vi "Read Autonomous Moves.vi"() -> ()   [LabVIEW 2012]
doc: "<B>Read Autonomous Moves</B> reads in a text file with a set of moves for the robot and executes those moves. \n\nThe text file must be in the following format:\nLine 1- X Joystick Value (double)\nLine 2- Y Joystick Value (double)\nLine 3- Movement Name (string of either \"right\", \"left\", \"forward\", \"reverse\", or \"stop\")\nLine 4- Encoder Ticks (double)\nLine 5- Empty\nRepeat"
uses:
  <vilib>/Rock Robotics/SystemInterfaces/DIO/FPGA_DIOChannel.ctl
  <vilib>/Rock Robotics/SystemInterfaces/DIO/FPGA_DIOPWMChannel.ctl
  <vilib>/Rock Robotics/SystemInterfaces/Typedef/FPGA_TypedefDigitalModule.ctl
  <vilib>/Rock Robotics/WPI/Counter/WPI_CounterDigitalInputToDigitalSource.vi
  <vilib>/Rock Robotics/WPI/RobotDrive/WPI_RobotDriveOpen2MotorWithJaguar.vi
  <vilib>/Rock Robotics/WPI/RobotDrive/WPI_RobotDriveArcadeDrive_Standard(NoSaturation).vi
  <vilib>/Rock Robotics/WPI/RobotDrive/WPI_RobotDriveArcadeDrive_RatioCurve.vi
panel:
  in  "Movement File Path":path=path "C:/RobotMoves.txt"
  in  "Right Motor (PWM Channel)":T1=enum."PWM 2"
  in  "Left Motor (PWM Channel)":T1
  in  "Encoder Channel 2":T2=enum."DIO 4"
  in  "Encoder Channel 1":T2=enum."DIO 3"
  # "Set these inputs before running."
  # "Wiring Diagram for Digital Sidecar connected to an NI 9403 in slot 4"
  # "Digital Sidecar"
  # "Power\nTerminals"
  # "Motor\nTerminals"
  # "PWM cable"
  # "This shows wiring for a Luminary Micro Jaguar speed controller.  The wiring is similar for a Victor speed controller.  For a Victor, you must also select the appropriate instance of the Motor Open VI on the diagram.  This is only the wiring for the Left Motor.  The Right Motor would be similarly wired to PWM Channel 2."
  # "Wiring Diagram for Digital Sidecar connected to an NI 9403"
  # "This shows wiring for a generic quadrature encoder.  Some encoders may have Gnd labeled as Com.  Some may have +5V labeled as +VDC."
  # "PWR"
  # "SIG"
  # "(-)"
  # "14\n13\n12\n11\n10\n9\n8\n7\n6\n5\n4\n3\n2\n1"
  # "Encoder"
  # "DIGITAL I/O"
  # "Index"
  # "Gnd"
  # "+5V"
  # "B"
  # "A"
  # "Digital Sidecar"
  # "PWR"
  # "SIG"
  # "(-)"
  # "+V"
  # "10"
  # "9"
  # "8"
  # "7"
  # "6"
  # "5"
  # "4"
  # "3"
  # "2"
  # "1"
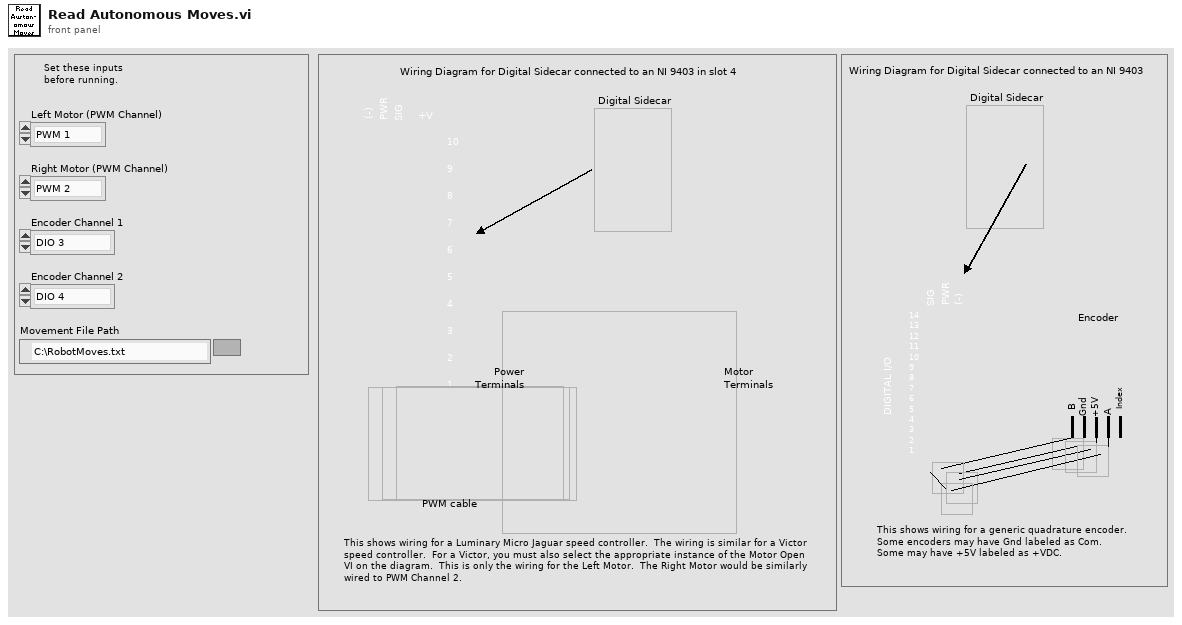
[diagram p1: front panel]
types:
  T1 = typedef "FPGA_DIOPWMChannel.ctl" = enum8{"PWM 1", "PWM 2", "PWM 3", "PWM 4", "PWM 5", "PWM 6", "PWM 7", "PWM 8", "PWM 9", "PWM 10", "Invalid"}
  T2 = typedef "FPGA_DIOChannel.ctl" = enum8{"DIO 1", "DIO 2", "DIO 3", "DIO 4", "DIO 5", "DIO 6", "DIO 7", "DIO 8", "DIO 9", "DIO 10", "DIO 11", "DIO 12", "DIO 13", "DIO 14", "Invalid"}
  T3 = typedef "FPGA_TypedefDigitalModule.ctl" = enum16{"Digital Module 1", "Digital Module 2"}
  T4 = typedef "WPI_DigitalInputDevRef.ctl" = cluster{"DevStatus":errorcluster, "DIO Channel":T2, "Digital Module":T3}
  T5 = typedef "FPGA_CounterEncoderSourceConvertionLVSourceType.ctl" = cluster{"DevStatus":errorcluster, "AnalogTriggerMode?":bool, "DigitalMode":cluster{"Digital Module":T3, "DIO Channel":T6}, "AnalogTriggerMode":cluster{"AnalogTriggerIndex":T7, "OutputType":T8}}
  T6 = typedef "FPGA_DIODigitalSourceChannel.ctl" = enum8{"DIO 1", "DIO 2", "DIO 3", "DIO 4", "DIO 5", "DIO 6", "DIO 7", "DIO 8", "DIO 9", "DIO 10", "DIO 11", "DIO 12", "DIO 13", "DIO 14", "Disabled"}
  T7 = typedef "FPGA_AnalogTriggerIndex.ctl" = enum8{"Trig 0", "Trig 1", "Trig 2", "Trig 3", "Trig 4", "Trig 5", "Trig 6", "Trig 7", "Invalid"}
  T8 = typedef "FPGA_AnalogTriggerOutType.ctl" = enum16{"InWindow", "TriggerState", "Rising", "Falling"}
  T9 = typedef "WPI_RobotDriveDevRef.ctl" = cluster{"DevStatus":errorcluster, "Motors[]":T10[], "Square Inputs":bool, "Max Output":dbl, "Isochronous":bool}
  T10 = typedef "WPI_MotorControlDeviceRef.ctl" = cluster{"DeviceStatus":errorcluster, "Type":enum16{"PWM", "CAN"}, "PWM":cluster{"Digital Module":T3, "PWM Channel":T1, "DeadBand":T11}, "CAN":cluster{"Device Number":u8, "Control Mode":T12, "Semaphore":T13, "Max Vout":dbl}, "Invert":bool, "TransformRef":T14, "InvTransformRef":T14}
  T11 = typedef "WPI_PWMDeadband.ctl" = cluster{"Name":string, "maxPositivePwm":i32, "minPositivePwm":i32, "centerPwm":i32, "maxNegativePwm":i32, "minNegativePwm":i32, "angularRange":u16}
  T12 = typedef "WPI_CANJaguar_ControlMode.ctl" = enum8{"Percent VBus", "Current", "Speed", "Position", "Voltage"}
  T13 = typedef "Semaphore RefNum" = refnum<k1>
  T14 = typedef "WPI_PWMTransform_ConPane.ctl" = refnum<vi>
  T15 = typedef "WPI_EncoderDevRef.ctl" = cluster{"DevStatus":errorcluster, "EncoderIndex":T16, "CounterIndex":T17, "DistancePerCount":dbl, "Decoding Type":T18}
  T16 = typedef "FPGA_EncoderIdx.ctl" = enum8{"Enc 0", "Enc 1", "Enc 2", "Enc 3", "Invalid"}
  T17 = typedef "FPGA_CounterCtrSystemIndex.ctl" = enum8{"Ctr 0", "Ctr 1", "Ctr 2", "Ctr 3", "Ctr 4", "Ctr 5", "Ctr 6", "Ctr 7", "Invalid"}
  T18 = typedef "WPI_EncoderType.ctl" = enum16{"1x", "2x", "4x"}
  T19 = cluster{"X Joystick Value":dbl, "Y Joystick Value":dbl, "Movement Name":string, "Ticks":dbl}[]
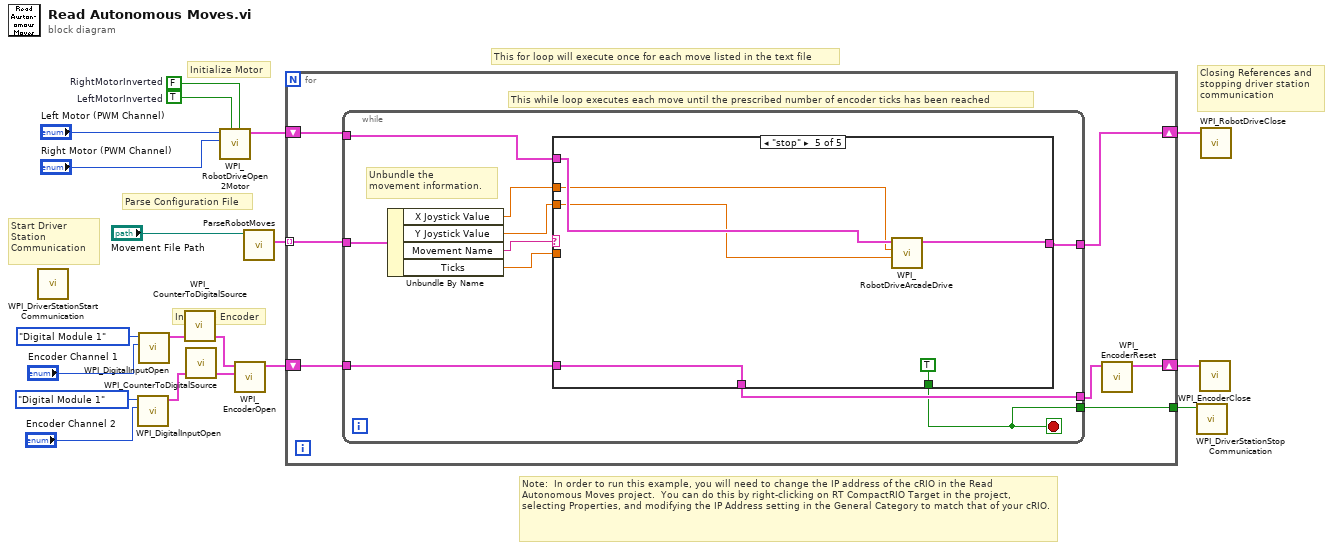
[diagram p0: block diagram]
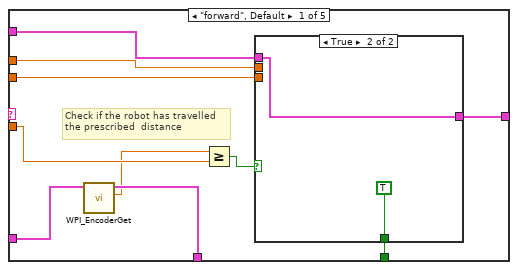
[diagram p2: hidden frame]
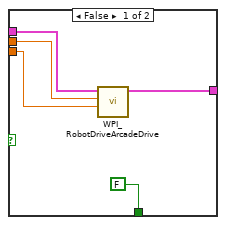
[diagram p3: hidden frame]
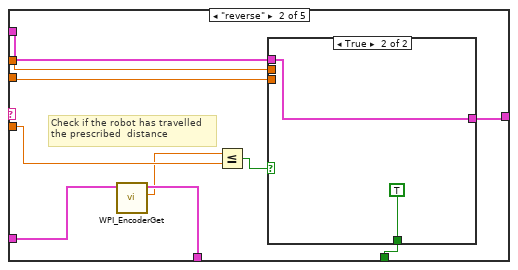
[diagram p4: hidden frame]
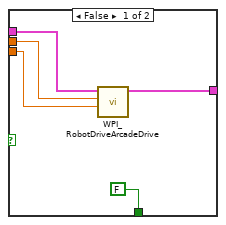
[diagram p5: hidden frame]
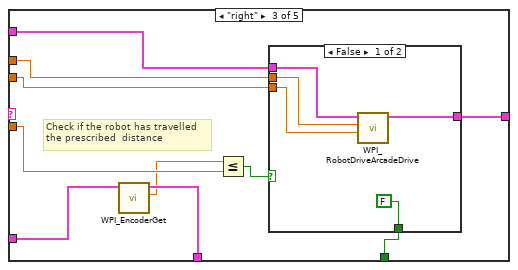
[diagram p6: hidden frame]
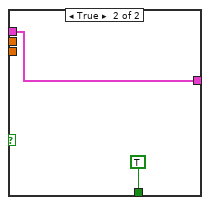
[diagram p7: hidden frame]
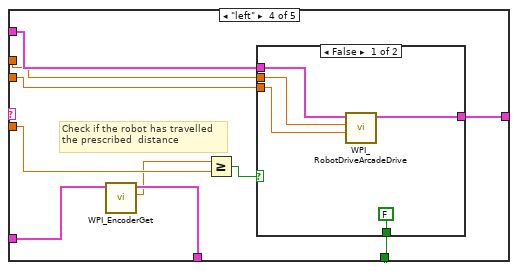
[diagram p8: hidden frame]
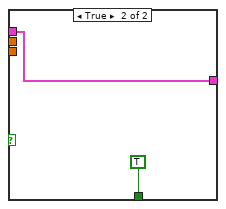
[diagram p9: hidden frame]
diagram:
  w7 = TRUE  # LeftMotorInverted
  w8 = FALSE  # RightMotorInverted
  # "Note:  In order to run this example, you will need to change the IP address of the cRIO in the Read Autonomous Moves project.  You can do this by right-clicking on RT CompactRIO Target in the project, selecting Properties, and modifying the IP Address setting in the General Category to match that of your cRIO."
  # "This for loop will execute once for each move listed in the text file"
  # "Start Driver\nStation \nCommunication"
  # "Closing References and\nstopping driver station\ncommunication"
  # "Parse Configuration File"
  # "Initialize Encoder"
  # "Initialize Motor"
  n1 = call <vilib>:"WPI_DriverStationStart Communication.vi"() -> ()  [unwired: 12 in]
  n2 = call <vilib>:"WPI_DigitalInputOpen.vi"("DIO Channel"="Encoder Channel 2", "Digital Module (Module 1)"=FPGA_TypedefDigitalModule."Digital Module 1") -> ("DigitalInputDevRef"=w16:T4)  [unwired: 8 in, 1 out]
  n3 = call <vilib>:"WPI_DigitalInputOpen.vi"("DIO Channel"="Encoder Channel 1", "Digital Module (Module 1)"=FPGA_TypedefDigitalModule."Digital Module 1") -> ("DigitalInputDevRef"=w17:T4)  [unwired: 8 in, 1 out]
  n4 = call-poly <vilib>:"WPI_CounterToDigitalSource.vi"("DigitalInputDevRef"=w17) -> ("Digital Source"=w14:T5)  [unwired: 6 in]
  n5 = call-poly <vilib>:"WPI_CounterToDigitalSource.vi"("DigitalInputDevRef"=w16) -> ("Digital Source"=w15:T5)  [unwired: 6 in]
  n6 = call-poly <vilib>:"WPI_RobotDriveOpen2Motor.vi"("Right Motor Inverted"=w8, "Left Motor Inverted"=w7, "Right Motor"="Right Motor (PWM Channel)", "Left Motor"="Left Motor (PWM Channel)") -> ("RobotDriveDevRef"=w4:T9)  [unwired: 1 in, 6 out]
  n7 = call <vilib>:"WPI_EncoderOpen.vi"("BSource"=w15, "ASource"=w14) -> ("EncoderDevRef"=w9:T15)  [unwired: 8 in, 1 out]
  n8 = call "ParseRobotMoves.vi"("file path (dialog if empty)"="Movement File Path") -> ("Array"=w18:T19)  [unwired: 10 in]
  n9 = for {
    tunnel: w18 -> [w23] mode=indexing
    shift-right: [w22] -> w2
    shift-left: w4 -> [w21]
    shift-right: [w24] -> w3
    shift-left: w9 -> [w26]
    tunnel: [w20] -> w1
    # "This while loop executes each move until the prescribed number of encoder ticks has been reached"
    n10 = while {
      tunnel: w21 -> [w36]
      tunnel: [w35] -> w22
      tunnel: w26 -> [w29]
      tunnel: [w28] -> w25
      tunnel: w23 -> [w34]
      tunnel: [w27] -> w20
      stop <- w27 stop-if-true
      # "Unbundle the \nmovement information."
      n11 = Unbundle By Name(w34) -> ("X Joystick Value"=w30:dbl, "Y Joystick Value"=w32:dbl, "Movement Name"=w33:string, "Ticks"=w31:dbl)
      n12 = case shown="\"stop\"" w33 {
        tunnel: w36 -> [w44 w62 w79 w95 w110]
        tunnel: w30 -> [w40 w61 w78 w91 w109]
        tunnel: w32 -> [w43 w60 w77 w94 w108]
        tunnel: w31 -> [w46 w59 w76 w93 _]
        tunnel: [w42 w57 w74 w96 w107] -> w35
        tunnel: [w41 w58 w75 w92 TRUE] -> w27
        tunnel: w29 -> [w39 w56 w73 w90 w105]
        tunnel: [w38 w55 w72 w89 w105] -> w28
        frame "forward", Default {
          # "Check if the robot has travelled\nthe prescribed  distance"
          n13 = call <vilib>:"WPI_EncoderGet.vi"("EncoderDevRef"=w39) -> ("Distance"=w37:dbl, "EncoderDevRef"=w38:T15)  [unwired: 5 in, 4 out]
          n14 = Greater Or Equal?(x=w37, y=w46) -> (x >= y?=w45:bool)
          n15 = case shown="True" w45 {
            tunnel: w44 -> [w51 w53]
            tunnel: w43 -> [w50 _]
            tunnel: [w49 w53] -> w42
            tunnel: [FALSE TRUE] -> w41
            tunnel: w40 -> [w47 _]
            frame False {
              n16 = call-poly <vilib>:"WPI_RobotDriveArcadeDrive.vi"("Y axis value"=w50, "X axis value"=w47, "RobotDriveDevRef"=w51) -> ("RobotDriveDevRef"=w49:T9)  [unwired: 1 in, 7 out]
            }
            frame True {
            }
          }
        }
        frame "reverse" {
          # "Check if the robot has travelled\nthe prescribed  distance"
          n17 = call <vilib>:"WPI_EncoderGet.vi"("EncoderDevRef"=w56) -> ("Distance"=w54:dbl, "EncoderDevRef"=w55:T15)  [unwired: 5 in, 4 out]
          n18 = Less Or Equal?(x=w54, y=w59) -> (x <= y?=w63:bool)
          n19 = case shown="True" w63 {
            tunnel: w62 -> [w68 w70]
            tunnel: w61 -> [w67 _]
            tunnel: w60 -> [w66 _]
            tunnel: [w65 w70] -> w57
            tunnel: [FALSE TRUE] -> w58
            frame False {
              n20 = call-poly <vilib>:"WPI_RobotDriveArcadeDrive.vi"("Y axis value"=w66, "X axis value"=w67, "RobotDriveDevRef"=w68) -> ("RobotDriveDevRef"=w65:T9)  [unwired: 1 in, 7 out]
            }
            frame True {
            }
          }
        }
        frame "right" {
          # "Check if the robot has travelled\nthe prescribed  distance"
          n21 = call <vilib>:"WPI_EncoderGet.vi"("EncoderDevRef"=w73) -> ("Distance"=w71:dbl, "EncoderDevRef"=w72:T15)  [unwired: 5 in, 4 out]
          n22 = Less Or Equal?(x=w71, y=w76) -> (x <= y?=w80:bool)
          n23 = case shown="False" w80 {
            tunnel: w79 -> [w85 w87]
            tunnel: w78 -> [w84 _]
            tunnel: w77 -> [w83 _]
            tunnel: [w82 w87] -> w74
            tunnel: [FALSE TRUE] -> w75
            frame False {
              n24 = call-poly <vilib>:"WPI_RobotDriveArcadeDrive.vi"("Y axis value (Speed)"=w83, "X axis value (Curve)"=w84, "RobotDriveDevRef"=w85) -> ("RobotDriveDevRef"=w82:T9)  [unwired: 2 in, 6 out]
            }
            frame True {
            }
          }
        }
        frame "left" {
          # "Check if the robot has travelled\nthe prescribed  distance"
          n25 = call <vilib>:"WPI_EncoderGet.vi"("EncoderDevRef"=w90) -> ("Distance"=w88:dbl, "EncoderDevRef"=w89:T15)  [unwired: 5 in, 4 out]
          n26 = Greater Or Equal?(x=w88, y=w93) -> (x >= y?=w97:bool)
          n27 = case shown="False" w97 {
            tunnel: w95 -> [w102 w104]
            tunnel: w91 -> [w101 _]
            tunnel: w94 -> [w100 _]
            tunnel: [w99 w104] -> w96
            tunnel: [FALSE TRUE] -> w92
            frame False {
              n28 = call-poly <vilib>:"WPI_RobotDriveArcadeDrive.vi"("Y axis value (Speed)"=w100, "X axis value (Curve)"=w101, "RobotDriveDevRef"=w102) -> ("RobotDriveDevRef"=w99:T9)  [unwired: 2 in, 6 out]
            }
            frame True {
            }
          }
        }
        frame "stop" {
          n29 = call-poly <vilib>:"WPI_RobotDriveArcadeDrive.vi"("Y axis value"=w108, "X axis value"=w109, "RobotDriveDevRef"=w110) -> ("RobotDriveDevRef"=w107:T9)  [unwired: 1 in, 7 out]
        }
      }
    }
    n30 = call <vilib>:"WPI_EncoderReset.vi"("EncoderDevRef"=w25) -> ("EncoderDevRef"=w24:T15)  [unwired: 9 in, 1 out]
  }
  n31 = call <vilib>:"WPI_DriverStationStop Communication.vi"("StopCommunication"=w1) -> ()  [unwired: 10 in, 1 out]
  n32 = call <vilib>:"WPI_EncoderClose.vi"("EncoderDevRef"=w3) -> ()  [unwired: 10 in, 1 out]
  n33 = call <vilib>:"WPI_RobotDriveClose.vi"("RobotDriveDevRef"=w2) -> ()  [unwired: 10 in, 1 out]
